vi "LaserCal-Initialize (meter).vi"(0 "Stimulus (meter)":T3, 7 "Options":T1, 11 "error in (no error)":errorcluster) -> (4 "Runtime State":T2={"AO Channels"=[], "Fs (Hz)"=100000.0, "Npts"=1, "conversion"=0.0}, 8 "Duty Cycle":dbl, 15 "error out":errorcluster)   [LabVIEW 2015]
uses:
  Typedefs/LaserCal-Meter Stimulus.ctl
  Typedefs/LaserCal-Control Mode.ctl
  Typedefs/LaserCal-Meter Runtime State.ctl
  Typedefs/LaserCal-Options.ctl
panel:
  in  "T (s)":dbl=1.0
  in  "Fs (Hz)":dbl=100000.0
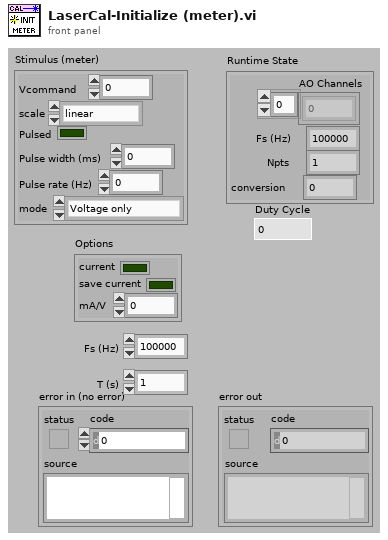
[diagram p1: front panel]
types:
  T1 = typedef "LaserCal-Options.ctl" = cluster{"current":bool, "save current":bool, "mA/V":dbl}
  T2 = typedef "LaserCal-Meter Runtime State.ctl" = cluster{"AO Channels":i32[], "Fs (Hz)":dbl, "Npts":i32, "conversion":dbl}
  T3 = typedef "LaserCal-Meter Stimulus.ctl" = cluster{"Vcommand":dbl, "scale":enum16{"linear", "dB"}, "Pulsed":bool, "Pulse width (ms)":dbl, "Pulse rate (Hz)":dbl, "mode":T4}
  T4 = typedef "LaserCal-Control Mode.ctl" = enum16{"Voltage only", "Voltage + Enable"}
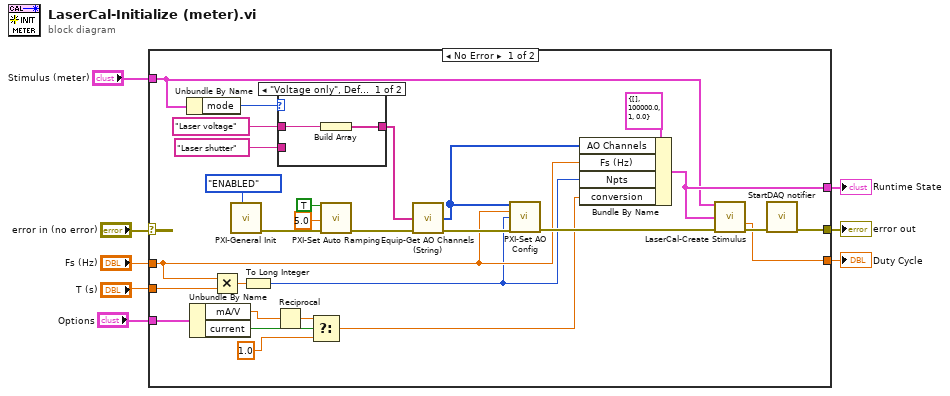
[diagram p0: block diagram]
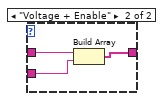
[diagram p2: hidden frame]
diagram:
  n1 = case shown="No Error" "error in (no error)" {
    selector: "error in (no error)" -> [_ w42]
    tunnel: [w31 w42] -> w7
    tunnel: "Fs (Hz)" -> [w27 _]
    tunnel: "T (s)" -> [w33 _]
    tunnel: "Stimulus (meter)" -> [w24 _]
    tunnel: [w25 _] -> w3
    tunnel: [w19 _] -> w2
    tunnel: "Options" -> [w14 _]
    frame No Error {
      n2 = Unbundle By Name(w24) -> ("mode"=w23:T4)
      n3 = Unbundle By Name(w14) -> ("mA/V"=w12:dbl, "current"=w13:bool)
      n4 = Multiply(x=w27, y=w33) -> (x*y=w32:dbl)
      n5 = call "PXI-General Init.vi"("Double Buffer Mode"=enum32{"OFF", "ENABLED", "FORCED"}."ENABLED") -> ("error out"=w18:errorcluster)  [unwired: 10 in]
      n6 = To Long Integer(number=w32) -> (32bit integer=w26:i32)
      n7 = Reciprocal(x=w12) -> (1/x=w9:dbl)
      n8 = case shown="\"Voltage only\", Default" w23 {
        tunnel: "Laser voltage" ("String") -> [w38 w41]
        tunnel: [w37 w40] -> w21
        tunnel: "Laser shutter" ("String") -> [_ w39]
        frame "Voltage only", Default {
          n9 = Build Array(w38) -> (w37:string[])
        }
        frame "Voltage + Enable" {
          n10 = Build Array(w41, w39) -> (w40:string[])
        }
      }
      n11 = Select(t=w9, s=w13, f=1.0) -> (s? t:f=w10:dbl)
      n12 = call "PXI-Set Auto Ramping.vi"("Auto ramp?"=TRUE, "Ramp duration (ms)"=5.0, "error in (no error)"=w18) -> ("error out"=w17:errorcluster)  [unwired: 12 in]
      n13 = call "Equip-Get AO Channels (String).vi"("Channel Names"=w21, "error in (no error)"=w17) -> ("AO Channels"=w28:i32[], "error out"=w34:errorcluster)  [unwired: 12 in]
      n14 = call "PXI-Set AO Config.vi"("AO Channels"=w28, "Sampling Rate (Hz)"=w27, "Buffer Size"=w26, "error in (no error)"=w34) -> ("error out"=w36:errorcluster)  [unwired: 11 in]
      n15 = Bundle By Name(cluster=T2 {"AO Channels"=[], "Fs (Hz)"=100000.0, "Npts"=1, "conversion"=0.0} ("Runtime State"), "AO Channels"=w28, "Fs (Hz)"=w27, "Npts"=w26, "conversion"=w10) -> (w25:T2)
      n16 = call "LaserCal-Create Stimulus.vi"("Stimulus"=w24, "Runtime State"=w25, "error in (no error)"=w36) -> ("Duty Cycle"=w19:dbl, "error out"=w30:errorcluster)  [unwired: 10 in, 1 out]
      n17 = call "StartDAQ notifier.vi"("error in (no error)"=w30) -> ("error out"=w31:errorcluster)  [unwired: 6 in]
    }
    frame Error {
    }
  }
  "error out" <- w7
  "Runtime State" <- w3
  "Duty Cycle" <- w2
